vi "AddSteppedVoltage.vi"(0 "deviceName":string, 1 "endVoltage":sgl, 2 "stepSize":sgl, 3 "isStartVoltageVsOCP":bool, 5 "channel":u8, 7 "repeats":u16=1, 8 "isAutoRange":bool=TRUE, 9 "startVoltage":sgl, 10 "approxMaxCurrent":sgl=inf, 11 "error in (no error)":errorcluster, 12 "samplingInterval":sgl, 13 "stepDuration":sgl, 14 "isEndVoltageVsOCP":bool) -> (15 "error out":errorcluster)   [LabVIEW 2018]
doc: "EXPORT void AisAddSteppedVoltage(const char* deviceName, uint8_t channel, uint16_t repeats, float startVoltage, float endVoltage, float samplingInterval, float stepSize, float stepDuration, bool isStartVoltageVsOCP, bool isEndVoltageVsOCP, float approxMaxCurrent, bool isAutoRange);"
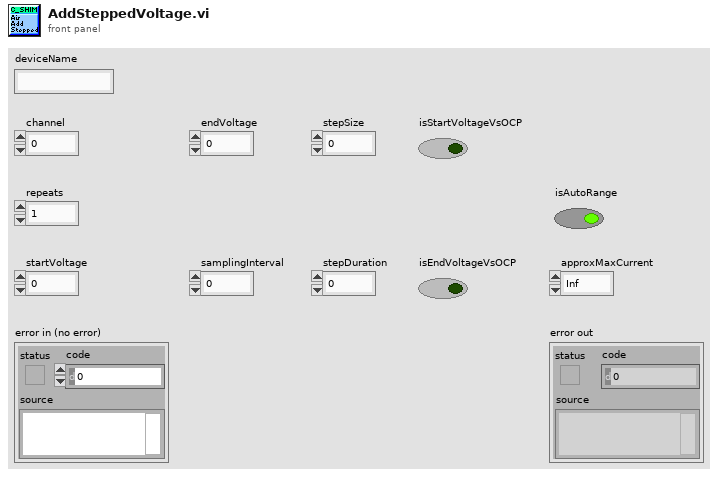
[diagram p1: front panel]
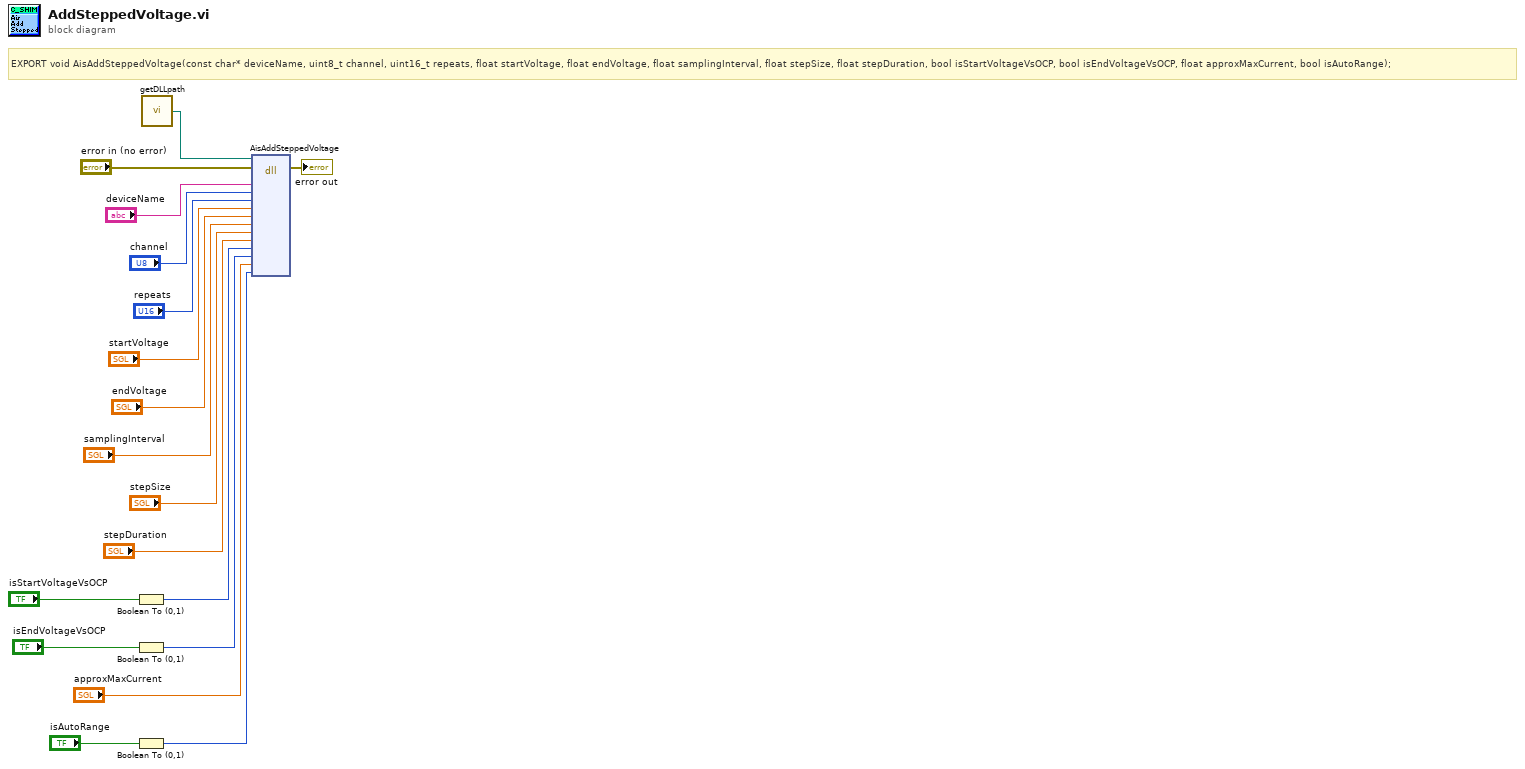
[diagram p0: block diagram]
diagram:
  # "EXPORT void AisAddSteppedVoltage(const char* deviceName, uint8_t channel, uint16_t repeats, float startVoltage, float endVoltage, float samplingInterval, float stepSize, float stepDuration, bool isStartVoltageVsOCP, bool isEndVoltageVsOCP, float approxMaxCurrent, bool isAutoRange);"
  n1 = Boolean To (0,1)(Boolean="isStartVoltageVsOCP") -> (0, 1=w9:i16)
  n2 = Boolean To (0,1)(Boolean="isEndVoltageVsOCP") -> (0, 1=w7:i16)
  n3 = Boolean To (0,1)(Boolean="isAutoRange") -> (0, 1=w4:i16)
  n4 = call "getDLLpath.vi"() -> ("DLL_Path"=w1:path)
  n5 = dll-call lib="?" fn="AisAddSteppedVoltage"(path in=w1, error in="error in (no error)", "deviceName"="deviceName", "channel"="channel", "repeats"="repeats", "startVoltage"="startVoltage", "endVoltage"="endVoltage", "samplingInterval"="samplingInterval", "stepSize"="stepSize", "stepDuration"="stepDuration", "isStartVoltageVsOCP"=w9, "isEndVoltageVsOCP"=w7, "approxMaxCurrent"="approxMaxCurrent", "isAutoRange"=w4) -> (error out=→"error out":errorcluster)  [unwired: 14 in, 1 out]
